vi "3Dzoomed.vi"() -> ()   [LabVIEW 2025]
uses:
  <vilib>/Analysis/1siggen.llb/Ramp Pattern by Samples.vi
  <vilib>/DAQmx/write.llb/DAQmx Write (Analog 1D Wfm NChan NSamp).vi
  <vilib>/DAQmx/read.llb/DAQmx Read (Counter 1D U32 1Chan NSamp).vi
  <vilib>/DAQmx/write.llb/DAQmx Write (Analog DBL 1Chan 1Samp).vi
  <vilib>/DAQmx/create/channels.llb/DAQmx Create Channel (AO-Voltage-Basic).vi
  <vilib>/DAQmx/configure/timing.llb/DAQmx Timing (Sample Clock).vi
  <vilib>/DAQmx/miscellaneous.llb/DAQmx Fill In Error Info.vi
  <vilib>/DAQmx/create/channels.llb/DAQmx Create Channel (CI-Count Edges).vi
  <vilib>/Analysis/NI_AALBase.lvlib
panel:
  in  "Enter length scanned (nm)":dbl
  in  "step-size in microns(depth)":dbl=0.1428 format="%#_13g"
  in  "Path":path
  in  "Number of z slices":i32
  out "transposed array":dbl[][](array[numeric])
  out "64bit integer":i64[](array[numeric])
  out "Intensity Graph":dbl[][](graph)
  out "Min Vy":dbl
  out "Max Vy":dbl
  out "Min Vx":dbl
  out "Max Vx":dbl
  out "appended array":dbl[][](array[numeric])
  in  "Dwell time (s)":dbl
  in  "new px":i32=128
  in  "Around desired spot":i32=128
  in  "Y coordinate":i32
  in  "X coordinate":i32
  in  "old px":i32=128
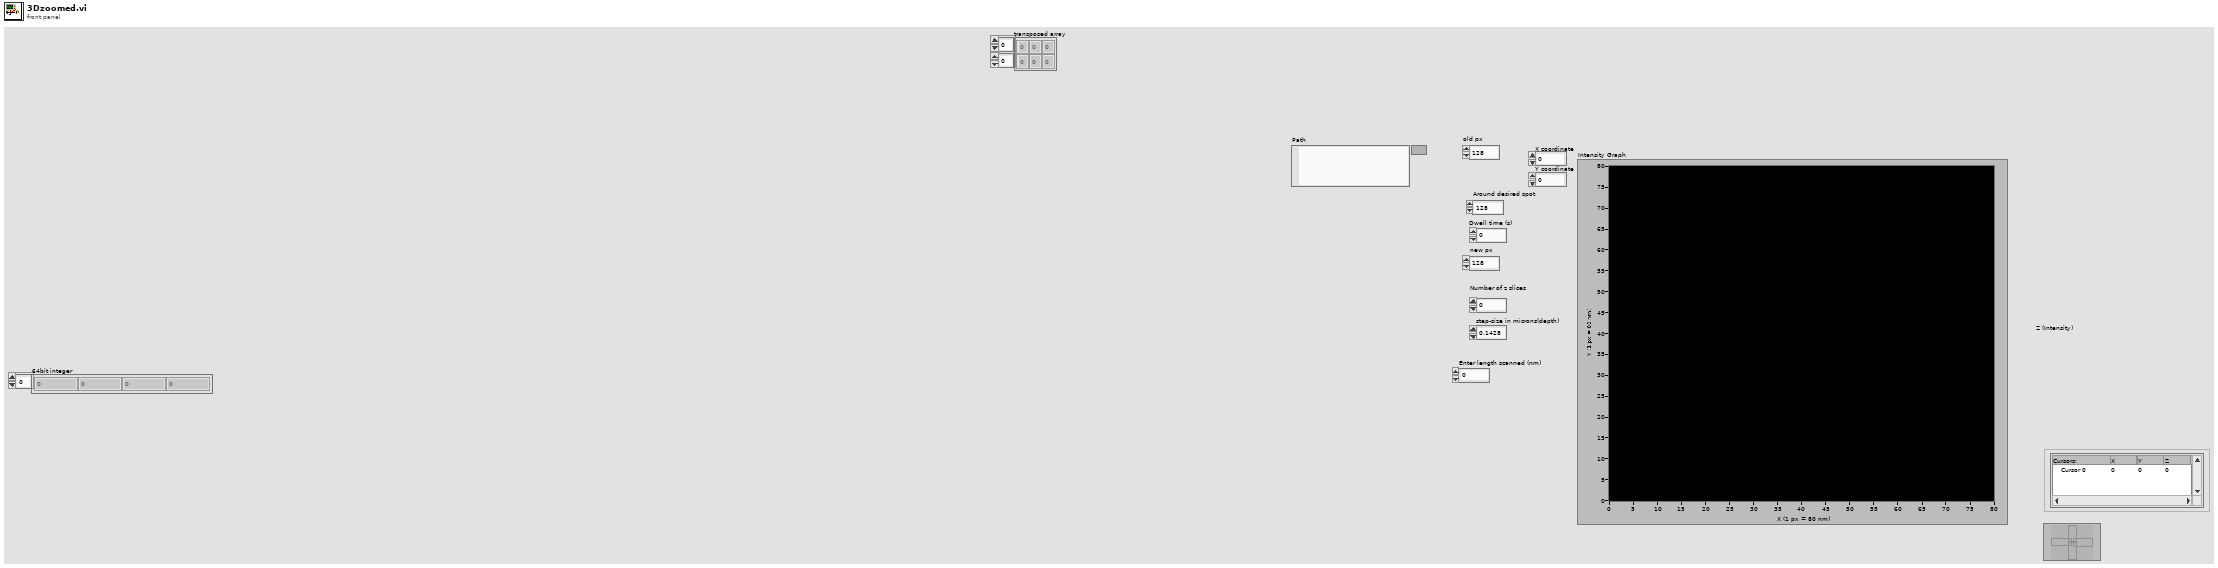
[diagram p1: front panel]
types:
  T1 = enum16{"big-endian, network order", "native, host order", "little-endian"}
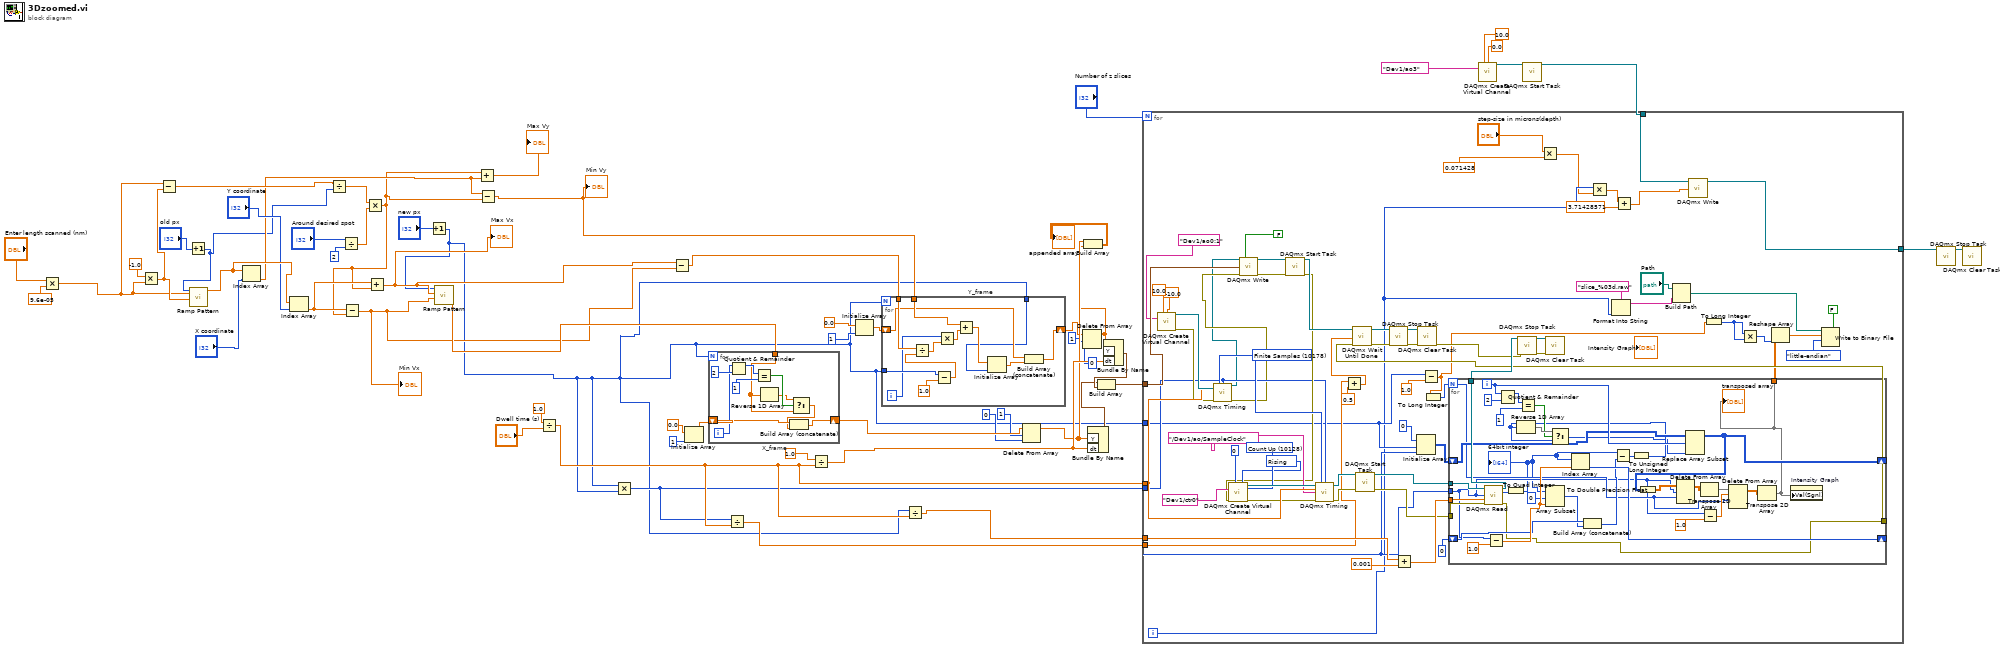
[diagram p0: block diagram]
diagram:
  n1 = Multiply(x="Enter length scanned (nm)", y=9.6e-05) -> (x*y=w3:dbl)
  n2 = Multiply(x=-1.0, y=w3) -> (x*y=w54:dbl)
  n3 = Subtract(x=w3, y=w54) -> (x-y=w53:dbl)
  n4 = Increment(x="old px") -> (x+1=w14:i32)
  n5 = call-poly <vilib>:"Ramp Pattern.vi"("start"=w54, "end"=w3, "samples"=w14) -> ("Ramp Pattern"=w58:dbl[])  [unwired: 7 in, 1 out]
  n6 = Index Array(array=w58, index="X coordinate") -> (element=w19:dbl)
  n7 = Index Array(array=w58, index="Y coordinate") -> (element=w21:dbl)
  n8 = Divide(x=w53, y=w14) -> (x/y=w52:dbl)
  n9 = Divide(x="Around desired spot", y=2) -> (x/y=w51:dbl)
  n10 = Multiply(x=w52, y=w51) -> (x*y=w18:dbl)
  n11 = Subtract(x=w21, y=w18) -> (x-y=w16:dbl)
  "Min Vx" <- w16
  n12 = Add(x=w21, y=w18) -> (x+y=w20:dbl)
  "Max Vx" <- w20
  n13 = Increment(x="new px") -> (x+1=w12:i32)
  n14 = call-poly <vilib>:"Ramp Pattern.vi"("start"=w16, "end"=w20, "samples"=w12) -> ("Ramp Pattern"=w22:dbl[])  [unwired: 7 in, 1 out]
  n15 = Add(x=w18, y=w19) -> (x+y=→"Max Vy":dbl)
  n16 = Subtract(x=w19, y=w18) -> (x-y=w15:dbl)
  "Min Vy" <- w15
  n17 = Divide(x=1.0, y="Dwell time (s)") -> (x/y=w28:dbl)
  n18 = Multiply(x=w12, y=w12) -> (x*y=w26:i32)
  n19 = Subtract(x=w20, y=w16) -> (x-y=w24:dbl)
  n20 = Initialize Array(0.0 ("element"), 1 ("dimension size")) -> (w43:dbl[])
  n21 = for "X_frame" {
    N: w12 -> [_]
    shift-right: [w69] -> w36
    shift-left: w43 -> [w70]
    tunnel: w22 -> [w63]
    i -> [w64]
    n22 = Quotient & Remainder(x=w64, y=2) -> (x-y*floor(x/y)=w67:i32)  [unwired: 1 out]
    n23 = Equal?(x=w67, y=1) -> (x = y?=w65:bool)
    n24 = Reverse 1D Array(array=w63) -> (reversed array=w62:dbl[])
    n25 = Select(t=w62, s=w65, f=w63) -> (s? t:f=w61:dbl[])
    n26 = Build Array (concatenate)(w70, w61) -> (w69:dbl[])
  }
  n27 = Divide(x=w26, y=w28) -> (x/y=w25:dbl)
  n28 = Divide(x=1.0, y=w28) -> (x/y=w45:dbl)
  n29 = Initialize Array(0.0 ("element"), 1 ("dimension size")) -> (w44:dbl[])
  n30 = for "Y_frame" {
    N: w12 -> [_]
    tunnel: w12 -> [w83]
    tunnel: w24 -> [w81]
    tunnel: w15 -> [w76]
    tunnel: w12 -> [w71]
    shift-right: [w72] -> w32
    shift-left: w44 -> [w73]
    i -> [w78]
    n31 = Subtract(x=w83, y=1.0) -> (x-y=w80:dbl)
    n32 = Divide(x=w81, y=w80) -> (x/y=w79:dbl)
    n33 = Multiply(x=w78, y=w79) -> (x*y=w77:dbl)
    n34 = Add(x=w76, y=w77) -> (x+y=w75:dbl)
    n35 = Initialize Array(w75, w71) -> (w74:dbl[])
    n36 = Build Array (concatenate)(w73, w74) -> (w72:dbl[])
  }
  n37 = Divide(x=w12, y=w28) -> (x/y=w27:dbl)
  n38 = Delete From Array "Delete From Array"(array=w36, length=1, index=0) -> (array with subset deleted=w33:dbl[])  [unwired: 1 out]
  n39 = Delete From Array "Delete From Array"(array=w32, length=1, index=0) -> (array with subset deleted=w29:dbl[])  [unwired: 1 out]
  n40 = Build Array(w33, w29) -> (→"appended array":dbl[][])
  n41 = Bundle By Name("Y"=w33, "dt"=w45) -> (w46:waveform(dbl))  [unwired: 1 in]
  n42 = Bundle By Name("Y"=w29, "dt"=w45) -> (w47:waveform(dbl))  [unwired: 1 in]
  n43 = Build Array(w46, w47) -> (w48:waveform(dbl)[])
  n44 = call-poly <vilib>:"DAQmx Create Virtual Channel.vi"("maximum value"=10.0, "minimum value"=0.0, "physical channels"=tag "Dev1/ao3") -> ("task out"=w11:refnum<k21>)  [unwired: 11 in, 1 out]
  n45 = call <vilib>:"DAQmx Start Task.vi"("task/channels in"=w11) -> ("task out"=w8:refnum<k21>)  [unwired: 13 in, 1 out]
  n46 = for {
    N: "Number of z slices" -> [_]
    tunnel: w48 -> [w140]
    tunnel: w28 -> [w130]
    tunnel: w27 -> [w127]
    tunnel: w26 -> [w114]
    tunnel: w25 -> [w113]
    tunnel: w12 -> [w109]
    tunnel: w8 -> [w104]
    tunnel: [w103] -> w6
    i -> [w92]
    w146 = 10178 items=["Finite Samples"=10178, "Continuous Samples"=10123, "Hardware Timed Single Point"=12522] ("Sample mode")
    w136 = 10280 items=["Rising"=10280, "Falling"=10171] ("edge")
    w137 = 10128 items=["Count Up"=10128, "Count Down"=10124, "Externally Controlled"=10326] ("count direction")
    n47 = call-poly <vilib>:"DAQmx Create Virtual Channel.vi"("maximum value"=10.0, "minimum value"=-10.0, "physical channels"="Dev1/ao0:1" ("Galvo mirror path")) -> ("task out"=w139:refnum<k21>, "error out"=w125:errorcluster)  [unwired: 11 in]
    n48 = call-poly <vilib>:"DAQmx Timing.vi"("task/channels in"=w139, "sample mode"=w146, "samples per channel"=w114, "rate"=w130, "error in"=w125) -> ("task out"=w105:refnum<k21>, "error out"=w106:errorcluster)  [unwired: 9 in]
    n49 = call-poly <vilib>:"DAQmx Write.vi"("task/channels in"=w105, "auto start"=FALSE, "data"=w140, "error in"=w106) -> ("task out"=w141:refnum<k21>, "error out"=w124:errorcluster)  [unwired: 9 in, 1 out]
    n50 = call <vilib>:"DAQmx Start Task.vi"("task/channels in"=w141, "error in"=w124) -> ("task out"=w148:refnum<k21>, "error out"=w121:errorcluster)  [unwired: 12 in]
    n51 = call-poly <vilib>:"DAQmx Create Virtual Channel.vi"("initial count"=u32 0, "count direction"=w137, "edge"=w136, "counter"="Dev1/ctr0" ("Counter path"), "error in"=w121) -> ("task out"=w143:refnum<k21>, "error out"=w123:errorcluster)  [unwired: 9 in]
    n52 = call-poly <vilib>:"DAQmx Timing.vi"("task/channels in"=w143, "sample mode"=w146, "samples per channel"=w114, "rate"=w130, "source"=tag "/Dev1/ao/SampleClock", "error in"=w123) -> ("task out"=w144:refnum<k21>, "error out"=w122:errorcluster)  [unwired: 8 in]
    n53 = Add(x=w113, y=0.5) -> (x+y=w111:dbl)
    n54 = call <vilib>:"DAQmx Start Task.vi"("task/channels in"=w144, "error in"=w122) -> ("task out"=w145:refnum<k21>, "error out"=w116:errorcluster)  [unwired: 12 in]
    n55 = Add(x=w127, y=0.001) -> (x+y=w131:dbl)
    n56 = Initialize Array(u32 0 ("element"), w109, w109) -> (w147:u32[][])
    n57 = Subtract(x=w109, y=1.0) -> (x-y=w87:dbl)
    n58 = To Long Integer(number=w87) -> (32bit integer=w88:i32)
    n59 = for {
      N: w88 -> [w158]
      tunnel: w109 -> [w155]
      tunnel: w131 -> [w185]
      tunnel: w145 -> [w184]
      shift-right: [w167] -> _
      shift-left: w147 -> [w170]
      tunnel: [w179] -> w126
      shift-right: [w176] -> _
      shift-left: u64 0 ("Numeric") -> [w174]
      tunnel: w116 -> [w165]
      tunnel: [w164] -> w115
      tunnel: [w152] -> w98
      i -> [w171]
      n60 = call-poly <vilib>:"DAQmx Read.vi"("task/channels in"=w184, "number of samples per channel"=w155, "timeout"=w185, "error in"=w165) -> ("task out"=w179:refnum<k21>, "data"=w166:u32[], "error out"=w164:errorcluster)  [unwired: 9 in]
      n61 = Subtract(x=w155, y=1.0) -> (x-y=w175:dbl)
      n62 = Quotient & Remainder(x=w171, y=2) -> (x-y*floor(x/y)=w182:i32)  [unwired: 1 out]
      n63 = To Quad Integer(1:w166) -> (0:w153:i64[])
      "64bit integer" <- w153
      n64 = Equal?(x=w182, y=1) -> (x = y?=w178:bool)
      n65 = Array Subset "Array Subset"(array=w153, index=0, length=w175) -> (w154:i64[])
      n66 = Index Array "Index Array"(array=w153, index=w175) -> (element=w176:i64)
      n67 = Build Array (concatenate) "Build Array"(w174, w154) -> (w173:u64[])
      n68 = Subtract(x=w153, y=w173) -> (x-y=w172:u64[])
      n69 = To Unsigned Long Integer(number=w172) -> (unsigned 32bit integer=w169:u32[])
      n70 = Reverse 1D Array(array=w169) -> (reversed array=w180:u32[])
      n71 = Select(t=w180, s=w178, f=w169) -> (s? t:f=w168:u32[])
      n72 = Replace Array Subset "Replace Array Subset"(array=w170, new element=w168, index (row)=w171) -> (w167:u32[][])  [unwired: 1 in]
      n73 = To Double Precision Float(number=w167) -> (double precision float=w163:dbl[][])
      n74 = Delete From Array(array=w163, length=w155, index (row)=w158) -> (array with subset deleted=w162:dbl[][])  [unwired: 1 in, 1 out]
      n75 = Transpose 2D Array(2D array=w162) -> (transposed array=w161:dbl[][])
      n76 = Subtract(x=w155, y=1.0) -> (x-y=w159:dbl)
      n77 = Delete From Array(array=w161, length=w159, index (row)=w158) -> (array with subset deleted=w157:dbl[][])  [unwired: 1 in, 1 out]
      n78 = Transpose 2D Array(2D array=w157) -> (transposed array=w152:dbl[][])
      "transposed array" <- w152
      n79 = property on="Intensity Graph" class="IntGraph (strict)"("Val(Sgnl)"=w152) -> ()  [unwired: 2 in, 2 out]
    }
    n80 = call <vilib>:"DAQmx Wait Until Done.vi"("task/channels in"=w148, "timeout (sec)"=w111, "error in"=w115) -> ("task out"=w149:refnum<k21>, "error out"=w120:errorcluster)  [unwired: 11 in]
    n81 = call <vilib>:"DAQmx Stop Task.vi"("task/channels in"=w149, "error in"=w120) -> ("task out"=w142:refnum<k21>, "error out"=w119:errorcluster)  [unwired: 12 in]
    n82 = call <vilib>:"DAQmx Clear Task.vi"("task in"=w142, "error in"=w119) -> ("error out"=w118:errorcluster)  [unwired: 13 in]
    n83 = call <vilib>:"DAQmx Stop Task.vi"("task/channels in"=w126, "error in"=w118) -> ("task out"=w150:refnum<k21>, "error out"=w117:errorcluster)  [unwired: 12 in]
    n84 = Multiply(x="step-size in microns(depth)", y=0.071428) -> (x*y=w86:dbl)
    n85 = call <vilib>:"DAQmx Clear Task.vi"("task in"=w150, "error in"=w117) -> ()  [unwired: 13 in, 1 out]
    n86 = Multiply(x=w92, y=w86) -> (x*y=w100:dbl)
    n87 = Format Into String(format string="slice_%03d.raw", w92) -> (resulting string=w90:string)  [unwired: 2 in, 1 out]
    n88 = Add(x=w100, y=3.71428571) -> (x+y=w102:dbl)
    n89 = Build Path(base path="Path", name or relative path=w90) -> (appended path=w94:path)
    n90 = call-poly <vilib>:"DAQmx Write.vi"("task/channels in"=w104, "data"=w102) -> ("task out"=w103:refnum<k21>)  [unwired: 11 in, 2 out]
    n91 = To Long Integer(number=w87) -> (32bit integer=w89:i32)
    n92 = Multiply(x=w89, y=w89) -> (x*y=w96:i32)
    n93 = Reshape Array(w98, w96) -> (w99:dbl[])
    n94 = Write to Binary File(file (use dialog)=w94, data=w99, 5:FALSE ("prepend array or string size? (T)"), 9:T1."little-endian" ("byte order (0:big-endian, network order)")) -> ()  [unwired: 2 in, 3 out]
  }
  n95 = call <vilib>:"DAQmx Stop Task.vi"("task/channels in"=w6) -> ("task out"=w7:refnum<k21>)  [unwired: 13 in, 1 out]
  n96 = call <vilib>:"DAQmx Clear Task.vi"("task in"=w7) -> ()  [unwired: 14 in, 1 out]
